vi "GetLengthInPulses.vi"(9 "pretrig":i32, 10 "revolutions":i32, 11 "speed ref channel":T1) -> (1 "pretrigger length in pulses":i32, 2 "pulses per rev":i32, 3 "total length in pulses":i32)   [LabVIEW 2017, in "DataAccumulator.lvlib"]
uses:
  <vilib>/addons/InsightCM/Devices/Shared/Common/DataAccumulator/DataAccumulator.lvlib
  <vilib>/addons/InsightCM/MessageBus/Base/controls/R2_Channel.ctl
  <vilib>/addons/InsightCM/MessageBus/Base/controls/KeyValuePair.ctl
  <vilib>/addons/InsightCM/MessageBus/Base/controls/Metric.ctl
  <vilib>/addons/InsightCM/Utilities/PropertyHelpers/PropertyHelpers.lvlib
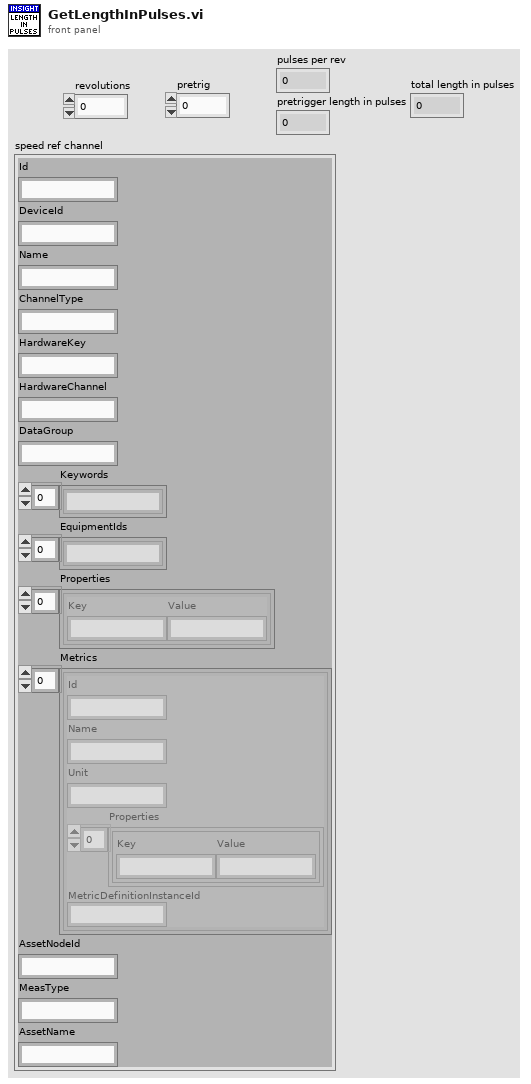
[diagram p1: front panel]
types:
  T1 = typedef "R2_Channel.ctl" = cluster{"Id":string, "DeviceId":string, "Name":string, "ChannelType":string, "HardwareKey":string, "HardwareChannel":string, "DataGroup":string, "Keywords":string[], "EquipmentIds":string[], "Properties":T2[], "Metrics":T3[], "AssetNodeId":string, "MeasType":string, "AssetName":string}
  T2 = typedef "KeyValuePair.ctl" = cluster{"Key":string, "Value":string}
  T3 = typedef "Metric.ctl" = cluster{"Id":string, "Name":string, "Unit":string, "Properties":T2[], "MetricDefinitionInstanceId":string}
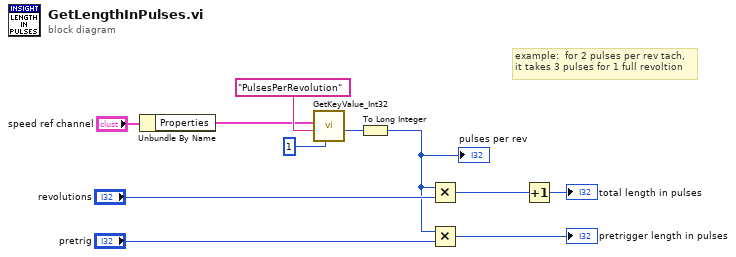
[diagram p0: block diagram]
diagram:
  # "example:  for 2 pulses per rev tach,\nit takes 3 pulses for 1 full revoltion"
  n1 = Unbundle By Name("speed ref channel") -> ("Properties"=w5:T2[])
  n2 = call <vilib>:"GetKeyValue_Int32.vi"("default"=1, "key"="PulsesPerRevolution" ("Name"), "key value pairs"=w5) -> ("value"=w6:i32)  [unwired: 6 in, 2 out]
  n3 = To Long Integer(number=w6) -> (32bit integer=w3:i32)
  "pulses per rev" <- w3
  n4 = Multiply(x=w3, y="revolutions") -> (x*y=w1:i32)
  n5 = Multiply(x=w3, y="pretrig") -> (x*y=→"pretrigger length in pulses":i32)
  n6 = Increment(x=w1) -> (x+1=→"total length in pulses":i32)
